vi "Create Test VIs.vi"(4 "error in":errorcluster) -> (0 "error out":errorcluster)   [LabVIEW 2025]
doc: "This VI creates all configured test VIs for unit testing. The configuration file <i>Test VI Definition.xml</i> must lie in the same folder as this VI."
uses:
  VI Definition--cluster.ctl
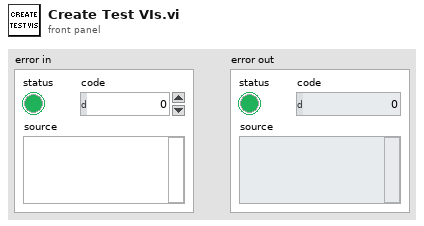
[diagram p1: front panel]
types:
  T1 = typedef "VI Definition--cluster.ctl" = cluster{"Name":string, "Description":string, "Numeric Indicators":cluster{"Labels":string[]}, "String Controls":cluster{"Labels":string[], "Default Values":string[]}, "Free Labels":cluster{"Text":string[]}, "Front Panel Labels":cluster{"Text":string[]}, "String Constants":cluster{"Text":string[]}}
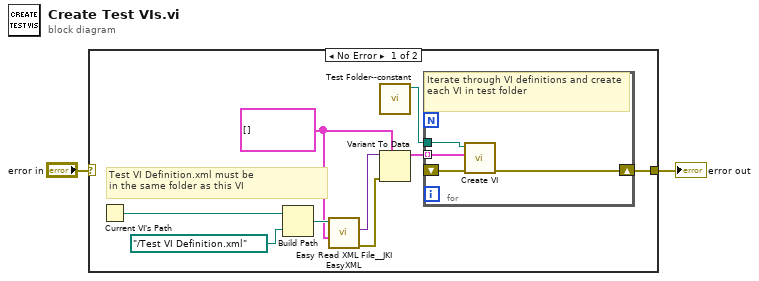
[diagram p0: block diagram]
diagram:
  n1 = case shown="No Error" "error in" {
    selector: "error in" -> [_ w16]
    tunnel: [w9 w16] -> w1
    frame No Error {
      w3 = T1[] [] ("Array")
      # "Test VI Definition.xml must be\nin the same folder as this VI"
      n2 = Current VI's Path() -> (path=w11:path)
      n3 = Build Path(base path=w11, name or relative path=path "../Test VI Definition.xml") -> (appended path=w6:path)
      n4 = call <vilib>:"Easy Read XML File__JKI EasyXML.vi"("LabVIEW Data (Type)"=w3, "XML File Path"=w6) -> ("error out"=w5:errorcluster, "LabVIEW Data"=w4:variant)  [unwired: 7 in, 1 out]
      n5 = call "Test Folder--constant.vi"() -> ("Test Folder"=w8:path)  [unwired: 7 in]
      n6 = Variant To Data(error in=w5, type=w3, Variant=w4) -> (data=w7:T1[])  [unwired: 1 out]
      n7 = for {
        tunnel: w8 -> [w15]
        tunnel: w7 -> [w14] mode=indexing
        shift-right: [w12] -> w9
        shift-left: _ -> [w13]
        # "Iterate through VI definitions and create each VI in test folder"
        n8 = call "Create VI.vi"("error in"=w13, "VI Definition"=w14, "Path"=w15) -> ("error out"=w12:errorcluster)  [unwired: 4 in]
      }
    }
    frame Error {
      # "Pass error without further action"
    }
  }
  "error out" <- w1
